vi "Query ID.vi"(8 "error in (no error)":errorcluster, 10 "Query String(*IDN?)":string="*IDN?", 11 "TCS in":refnum<class "TCS.lvclass">) -> (0 "error out":errorcluster, 2 "ID  string":string, 3 "TCS out":refnum<class "TCS.lvclass">)   [LabVIEW 2013, in "TCS.lvclass"]
uses:
  Lib.llb/TCS.lvclass
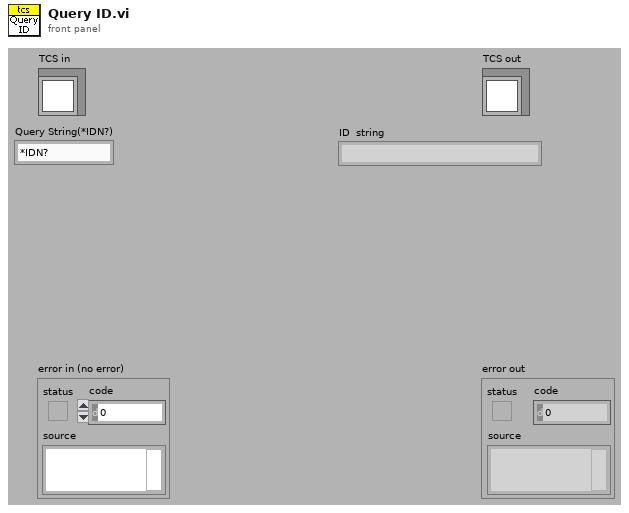
[diagram p1: front panel]
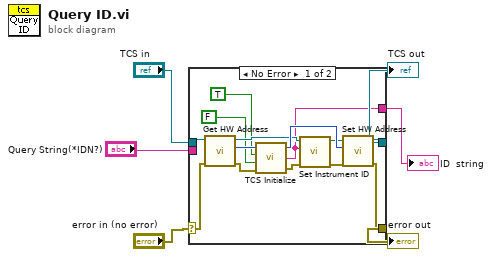
[diagram p0: block diagram]
diagram:
  n1 = case shown="No Error" "error in (no error)" {
    selector: "error in (no error)" -> [w14 w21]
    tunnel: [w15 w21] -> w6
    tunnel: [w16 w22] -> w5
    tunnel: "Query String(*IDN?)" -> [_ _]
    tunnel: "TCS in" -> [w20 w22]
    tunnel: [w9 _] -> w1
    frame No Error {
      n2 = call-dynamic "Get HW Address.vi"("error in (no error)"=w14, "CS.lvclass in"=w20) -> ("error out"=w18:errorcluster, "HW Address"=w19:u32, "CS.lvclass out"=w13:refnum<class "TCS.lvclass">)  [unwired: 7 in]
      n3 = call "TCS Initialize.vi"("port number (1:com2)"=w19, "ID query"=TRUE, "reset"=FALSE, "error in (no error)"=w18) -> ("port number out"=w17:i32, "ID string retrieved from TCS"=w9:string, "error out"=w10:errorcluster)  [unwired: 1 in]
      n4 = call-dynamic "Set Instrument ID.vi"("error in (no error)"=w10, "Instrument ID"=w9, "CS.lvclass in"=w13) -> ("error out"=w11:errorcluster, "CS.lvclass out"=w12:refnum<class "TCS.lvclass">)  [unwired: 7 in]
      n5 = call-dynamic "Set HW Address.vi"("error in (no error)"=w11, "HW Address"=w17, "CS.lvclass in"=w12) -> ("error out"=w15:errorcluster, "CS.lvclass out"=w16:refnum<class "TCS.lvclass">)  [unwired: 7 in]
    }
    frame Error {
    }
  }
  "error out" <- w6
  "TCS out" <- w5
  "ID  string" <- w1
